vi "find glyph data by name.vi"(8 "error in":errorcluster, 9 "overlay":string, 10 "name":string, 11 "glyph manager in":T2) -> (0 "error out":errorcluster, 1 "image data":T1, 2 "symbol index":i32, 3 "glyph manager out":T2)   [LabVIEW 2025, in "CEF.lvlib"]
doc: "Copyright 2017 National Instruments Corporation\n\nLicensed under the Apache License, Version 2.0 (the \"License\"); you may not use this file except in compliance with the License. You may obtain a copy of the License at http://www.apache.org/licenses/LICENSE-2.0\nUnless required by applicable law or agreed to in writing, software distributed under the License is distributed on an \"AS IS\" BASIS, WITHOUT WARRANTIES OR CONDITIONS OF ANY KIND, either express or implied. See the License for the specific language governing permissions and limitations under the License."
uses:
  CEF.lvlib
  glyph manager.ctl
  <vilib>/picture/picture.llb/imagedata.ctl
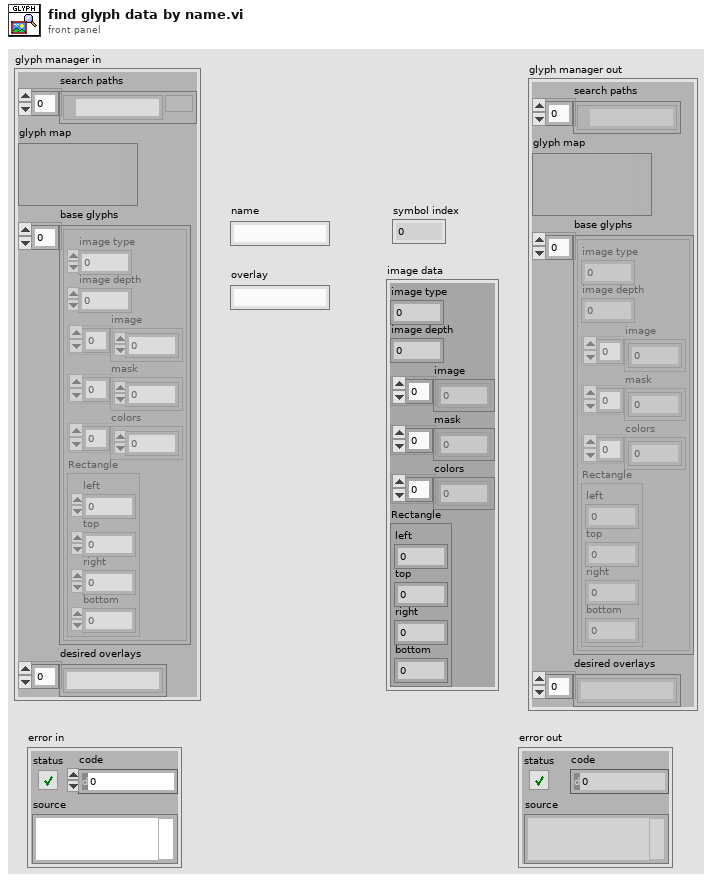
[diagram p1: front panel]
types:
  T1 = typedef "imagedata.ctl" = cluster{"image type":i32, "image depth":i32, "image":u8[], "mask":u8[], "colors":u32[], "Rectangle":cluster{"left":i16, "top":i16, "right":i16, "bottom":i16}}
  T2 = typedef "CEF.lvlib/glyph manager.ctl" = cluster{"search paths":path[], "glyph map":variant, "base glyphs":T1[], "desired overlays":string[]}
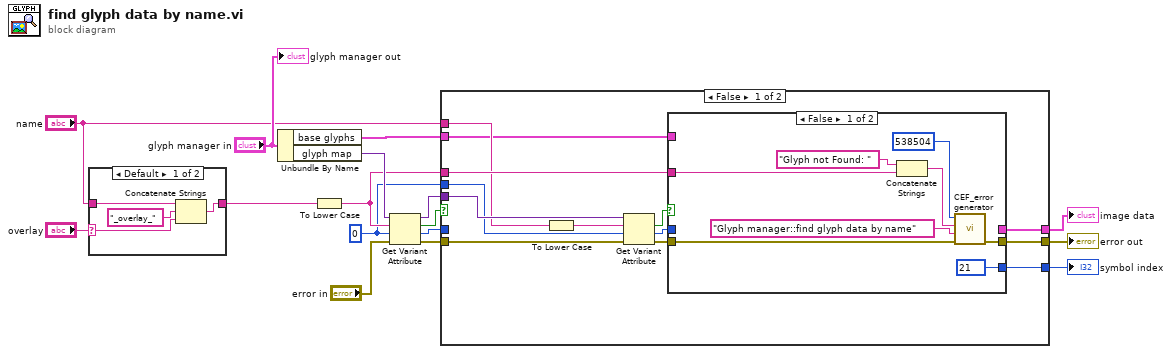
[diagram p0: block diagram]
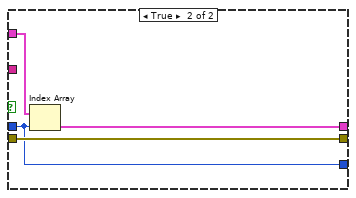
[diagram p3: hidden frame]
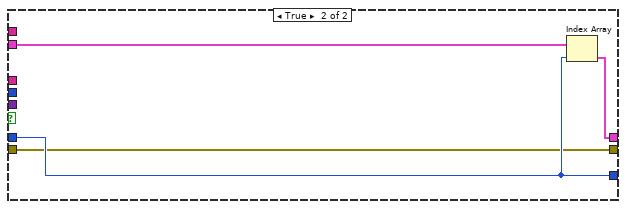
[diagram p4: hidden frame]
diagram:
  w1 = 0
  n1 = case shown="Default" "overlay" {
    selector: "overlay" -> [w17 _]
    tunnel: [w19 w21] -> w5
    tunnel: "name" -> [w18 w21]
    frame Default {
      n2 = Concatenate Strings(w18, "_overlay_" ("string"), w17) -> (w19:string)
    }
    frame "" {
    }
  }
  n3 = Unbundle By Name("glyph manager in") -> ("base glyphs"=w11:T1[], "glyph map"=w15:variant)
  n4 = To Lower Case(string=w5) -> (all lower case string=w6:string)
  n5 = Get Variant Attribute(Variant=w15, name=w6, default value (empty Variant)=w1, error in="error in") -> (duplicate Variant=w3:variant, found=w13:bool, value=w9:i32, error out=w12:errorcluster)
  n6 = case shown="False" w13 {
    tunnel: w12 -> [w34 w47]
    tunnel: w11 -> [w24 w50]
    tunnel: [w23 w49] -> w10
    tunnel: w9 -> [_ w48]
    tunnel: [w31 w48] -> w8
    tunnel: [w33 w47] -> w7
    tunnel: w6 -> [w32 _]
    tunnel: w3 -> [w29 _]
    tunnel: "name" -> [w28 _]
    tunnel: w1 -> [w27 _]
    frame False {
      n7 = To Lower Case(string=w28) -> (all lower case string=w22:string)
      n8 = Get Variant Attribute(Variant=w29, name=w22, default value (empty Variant)=w27, error in=w34) -> (found=w26:bool, value=w25:i32, error out=w30:errorcluster)  [unwired: 1 out]
      n9 = case shown="False" w26 {
        tunnel: [w42 w44] -> w33
        tunnel: w32 -> [w37 _]
        tunnel: [21 w43] -> w31
        tunnel: w30 -> [w35 w44]
        tunnel: w25 -> [_ w43]
        tunnel: w24 -> [_ w46]
        tunnel: [_ w45] -> w23
        frame False {
          n10 = Concatenate Strings("Glyph not Found: " ("string"), w37) -> (w38:string)
          n11 = call "CEF_error generator.vi"("error in"=w35, "source"="Glyph manager::find glyph data by name", "append error message"=w38, "error code (0)"=538504 ("code")) -> ("error out"=w42:errorcluster)  [unwired: 5 in]
        }
        frame True {
          n12 = Index Array(array=w46, index=w43) -> (element=w45:T1)
        }
      }
    }
    frame True {
      n13 = Index Array(array=w50, index=w48) -> (element=w49:T1)
    }
  }
  "error out" <- w7
  "image data" <- w10
  "symbol index" <- w8
  "glyph manager out" <- "glyph manager in"
